vi "Generate Simulated Cars.vi"() -> ()   [LabVIEW 2017]
panel:
  in  "# Cars":i32=10
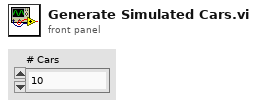
[diagram p1: front panel]
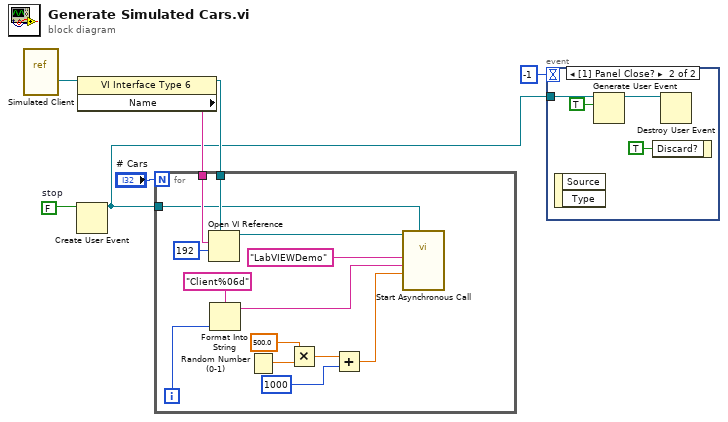
[diagram p0: block diagram]
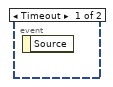
[diagram p2: hidden frame]
diagram:
  w3 = FALSE  # stop
  n1 = vi-ref "Simulated Client.vi"() -> (w6:refnum<vi>)
  n2 = Create User Event(user event datatype=w3) -> (user event=w1:refnum<user-event>)  [unwired: 1 in, 1 out]
  n3 = property class="VI Interface Type 6"(reference=w6) -> (reference out=w4:refnum<vi>, "Name"=w5:string)  [unwired: 1 in, 1 out]
  n4 = for {
    N: "# Cars" -> [_]
    tunnel: w5 -> [w20]
    tunnel: w4 -> [w18]
    tunnel: w1 -> [w17]
    i -> [w15]
    n5 = Open VI Reference(type specifier VI Refnum (for type only)=w18, vi path=w20, options=192) -> (vi reference=w19:refnum<vi>)  [unwired: 3 in, 1 out]
    n6 = Format Into String(format string="Client%06d", w15) -> (resulting string=w14:string)  [unwired: 2 in, 1 out]
    n7 = Random Number (0-1)() -> (number: 0 to 1=w12:dbl)
    n8 = Multiply(x=500.0, y=w12) -> (x*y=w10:dbl)
    n9 = Add(x=w10, y=1000 ("period (ms)")) -> (x+y=w8:dbl)
    n10 = call-by-ref "Start Asynchronous Call"(reference=w19, "Stop Signal"=w17, "period (ms)"=w8, "Client Name"=w14, "project namespace"="LabVIEWDemo") -> ()  [unwired: 9 in, 2 out]
  }
  n11 = event shown="[1] Panel Close?" {
    selector: _ -> [_ _]
    dyn-events: _ -> [_ _]
    timeout: -1 -> [_ _]
    tunnel: w1 -> [_ w23]
    event Timeout {
      n12 = event-data() -> ()  [unwired: 1 in, 1 out]
    }
    event Panel Close? {
      n13 = event-data() -> ()  [unwired: 1 in, 2 out]
      n14 = Generate User Event(user event=w23, event data cluster=TRUE ("event data")) -> (user event out=w24:refnum<user-event>)  [unwired: 2 in, 1 out]
      n15 = event-data("Discard?"=TRUE) -> ()  [unwired: 1 in, 1 out]
      n16 = Destroy User Event(user event=w24) -> ()  [unwired: 1 in, 1 out]
    }
  }
